vi "CRC.vi"(8 "Size":u8, 9 "Offset":i16, 11 "Data":u8[](array[numeric])) -> (0 "CRC Lo":u8, 3 "CRC Hi":u8)   [LabVIEW 2018]
uses:
  <vilib>/rvi/DesktopExecutionNode/Execution/niFpgaDEN_Execute.vi
  <vilib>/rvi/DesktopExecutionNode/DesktopExecutionNode.xnode
panel:
  # "Calculates ModBus 16 bit CRC\n\nInput is array of uint8 values. Output is two\nuint8 values, representing CRC."
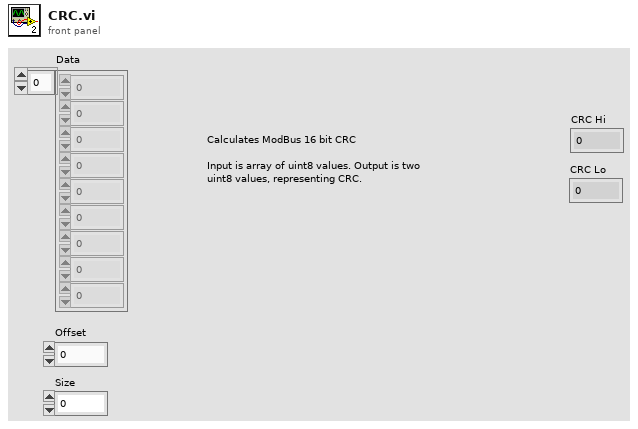
[diagram p1: front panel]
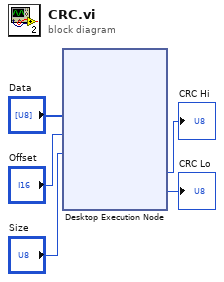
[diagram p0: block diagram]
diagram:
  n1 = xnode "Desktop Execution Node"("Data"="Data", "Offset"="Offset", "Size"="Size") -> ("CRC Hi"=→"CRC Hi":u8, "CRC Lo"=→"CRC Lo":u8)  [unwired: 1 in, 1 out]
